vi "createTestObject.vi"(11 "Data in":T1={"Report.lvclass"=refnum, "Norm"="", "last State"=enum."Initialize", "Norm ID"=0, "EMTestCWS500N.lvclass"=refnum, "CEG4500.lvclass"=refnum, "Tektronix RSA5106A.lvclass"=refnum, "erfolgreich"=FALSE, "Device Enum"=enum."emTestCWS500N", "Test Enum"=enum."ESD", "debug"=FALSE, "tab"=enum."Hauptmenü", "ESD Pistol.lvclass"=refnum, "SubPnl Refnum"=refnum, "TabCtl Refnum"=refnum, "ButtonsEinblenden?"=FALSE, "VKey"=enum."ASCII", "last Test"=refnum}) -> (3 "Data out":T1={"Report.lvclass"=refnum, "Norm"="", "last State"=enum."Initialize", "Norm ID"=0, "EMTestCWS500N.lvclass"=refnum, "CEG4500.lvclass"=refnum, "Tektronix RSA5106A.lvclass"=refnum, "erfolgreich"=FALSE, "Device Enum"=enum."emTestCWS500N", "Test Enum"=enum."ESD", "debug"=FALSE, "tab"=enum."Hauptmenü", "ESD Pistol.lvclass"=refnum, "SubPnl Refnum"=refnum, "TabCtl Refnum"=refnum, "ButtonsEinblenden?"=FALSE, "VKey"=enum."ASCII", "last Test"=refnum})   [LabVIEW 2013]
uses:
  Main/controls/Data.ctl
  classes/Datastructure/Report/Report.lvclass
  classes/Devices/emTestCWS500N/EMTestCWS500N.lvclass
  classes/Devices/CEG4500/CEG4500.lvclass
  classes/Devices/Tektronix RSA5106A/Tektronix RSA5106A.lvclass
  ESD Pistol.lvclass
  classes/Datastructure/Test/Test.lvclass
  Main/controls/State.ctl
  classes/Devices/DeviceInterface/Devices.ctl
  classes/Tests/TestInterface/Tests.ctl
  Tabs.ctl
  <vilib>/event_ctls.llb/eventvkey.ctl
  classes/Tests/TestInterface/TestInterface.lvclass
  classes/Devices/DeviceInterface/DeviceInterface.lvclass
  classes/Tests/Stoeraussendung/Stoeraussendung.lvclass
  classes/Tests/Burst/Burst.lvclass
  classes/Tests/Surge/Surge.lvclass
  classes/Tests/Spannungseinbruch/Spannungseinbruch.lvclass
  classes/Tests/HF-Felder/HF-Felder.lvclass
  classes/Tests/ESD/ESD.lvclass
panel:
  out "error out":errorcluster
  in  "error in":errorcluster
types:
  T1 = typedef "Data.ctl" = cluster{"Report.lvclass":refnum<class "Report.lvclass">, "Norm":string, "last State":T2, "Norm ID":i32, "EMTestCWS500N.lvclass":refnum<class "EMTestCWS500N.lvclass">, "CEG4500.lvclass":refnum<class "CEG4500.lvclass">, "Tektronix RSA5106A.lvclass":refnum<class "Tektronix RSA5106A.lvclass">, "erfolgreich":bool, "Device Enum":T3, "Test Enum":T4, "debug":bool, "tab":T5, "ESD Pistol.lvclass":refnum<class "ESD Pistol.lvclass">, "SubPnl Refnum":refnum<vi>, "TabCtl Refnum":refnum<vi>, "ButtonsEinblenden?":bool, "VKey":T6, "last Test":refnum<class "Test.lvclass">}
  T2 = typedef "State.ctl" = enum16{"create Pdf", "edit Report", "load Report", "save Report", "do Test", "CDN Kalibrierung", "enter Report Parameters", "new Test", "Protokoll", "read Tree", "update Tree", "Fehler", "Initialize", "Wait for Event", "Exit"}
  T3 = typedef "Devices.ctl" = enum16{"unbekannt", "ESD Pistol", "Tektronix RSA5106A", "emTestCWS500N", "CEG-4500"}
  T4 = typedef "Tests.ctl" = enum16{"unbekannt", "Störaussendung", "Burst", "ESD", "Surge", "Spannungseinbruch", "HF-Felder"}
  T5 = typedef "Tabs.ctl" = enum32{"Hauptmenü", "Prüfbericht", "Einstellungen"}
  T6 = typedef "eventvkey.ctl" = enum16{"ASCII", "Enter", "Return", "Shift", "Ctrl", "Alt", "Cmd", "Opt", "Caps", "NumLock", "Clear", "Break", "Up", "Down", "Left", "Right", "Insert", "Delete", "Home", "End", "PageUp", "PageDown", "Escape", "Help", "Pause", "ScrollLock", "F1", "F2", "F3", "F4", "F5", "F6", "F7", "F8", "F9", "F10", "F11", "F12", "F13", "F14", "F15", "F16", "F17", "F18", "F19", "F20", "F21", "F22", "F23", "F24", "Play", "VolumeUp", "VolumeDown", "Mute", "Two Byte Char"}
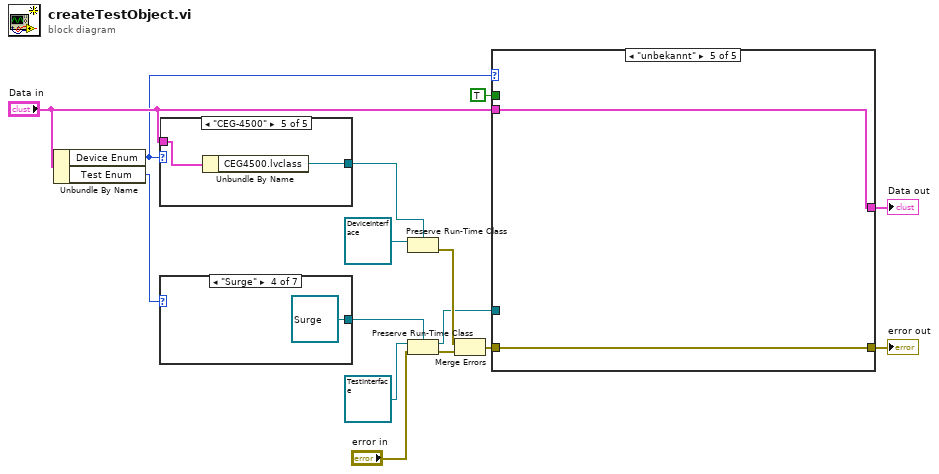
[diagram p0: block diagram]
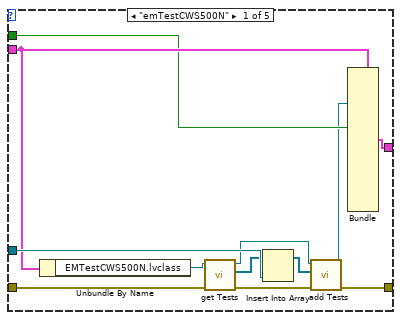
[diagram p2: hidden frame]
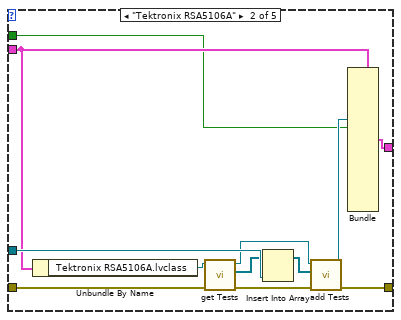
[diagram p3: hidden frame]
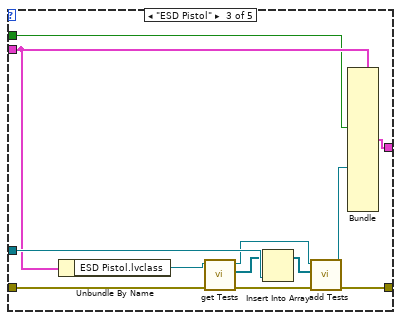
[diagram p4: hidden frame]
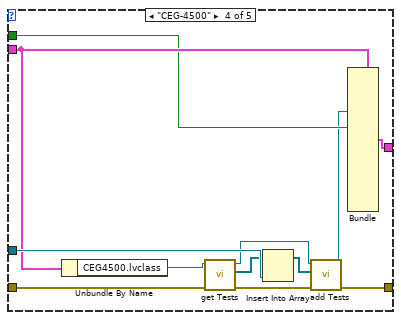
[diagram p5: hidden frame]
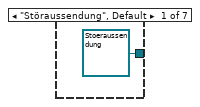
[diagram p6: hidden frame]
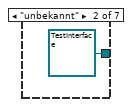
[diagram p7: hidden frame]
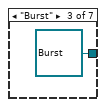
[diagram p8: hidden frame]
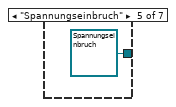
[diagram p9: hidden frame]
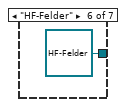
[diagram p10: hidden frame]
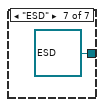
[diagram p11: hidden frame]
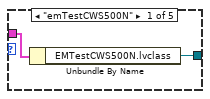
[diagram p12: hidden frame]
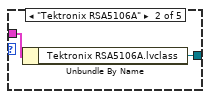
[diagram p13: hidden frame]
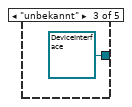
[diagram p14: hidden frame]
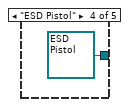
[diagram p15: hidden frame]
diagram:
  n1 = Unbundle By Name("Data in") -> ("Device Enum"=w12:T3, "Test Enum"=w11:T4)
  n2 = case shown="\"CEG-4500\"" w12 {
    tunnel: [w16 w18 refnum<class "DeviceInterface.lvclass"> refnum ("Tektronix RSA5106A.lvclass") refnum<class "ESD Pistol.lvclass"> refnum ("ESD Pistol.lvclass") w22] -> w9
    tunnel: "Data in" -> [w17 w19 _ _ w23]
    frame "emTestCWS500N" {
      n3 = Unbundle By Name(w17) -> ("EMTestCWS500N.lvclass"=w16:refnum<class "EMTestCWS500N.lvclass">)
    }
    frame "Tektronix RSA5106A" {
      n4 = Unbundle By Name(w19) -> ("Tektronix RSA5106A.lvclass"=w18:refnum<class "Tektronix RSA5106A.lvclass">)
    }
    frame "unbekannt" {
    }
    frame "ESD Pistol" {
    }
    frame "CEG-4500" {
      n5 = Unbundle By Name(w23) -> ("CEG4500.lvclass"=w22:refnum<class "CEG4500.lvclass">)
    }
  }
  n6 = case shown="\"Surge\"" w11 {
    tunnel: [refnum<class "Stoeraussendung.lvclass"> refnum ("Störaussendung.lvclass") refnum<class "TestInterface.lvclass"> refnum ("Burst.lvclass") refnum<class "Burst.lvclass"> refnum ("Burst.lvclass") refnum<class "Surge.lvclass"> refnum ("Surge.lvclass") refnum<class "Spannungseinbruch.lvclass"> refnum ("Spannungseinbruch.lvclass") refnum<class "HF-Felder.lvclass"> refnum ("HF-Felder.lvclass") refnum<class "ESD.lvclass"> refnum ("ESD.lvclass")] -> w6
    frame "Störaussendung", Default {
    }
    frame "unbekannt" {
    }
    frame "Burst" {
    }
    frame "Surge" {
    }
    frame "Spannungseinbruch" {
    }
    frame "HF-Felder" {
    }
    frame "ESD" {
    }
  }
  n7 = Preserve Run-Time Class(object in=refnum<class "DeviceInterface.lvclass"> refnum ("DeviceInterface.lvclass"), 2:w9) -> (error out=w8:errorcluster)  [unwired: 1 in, 1 out]
  n8 = Preserve Run-Time Class(object in=refnum<class "TestInterface.lvclass"> refnum ("TestInterface.lvclass"), error in="error in", 2:w6) -> (object out=w3:refnum<class "TestInterface.lvclass">, error out=w7:errorcluster)
  n9 = Merge Errors(w8, w7) -> (w2:errorcluster)
  n10 = case shown="\"unbekannt\"" w12 {
    tunnel: TRUE ("erfolgreich") -> [w32 w43 w56 w68 _]
    tunnel: w3 -> [w42 w54 w66 w78 _]
    tunnel: w2 -> [w41 w53 w65 w77 w80]
    tunnel: [w40 w52 w64 w76 w80] -> w13
    tunnel: [w39 w51 w63 w75 w79] -> w14
    tunnel: "Data in" -> [w38 w50 w62 w74 w79]
    frame "emTestCWS500N" {
      n11 = Unbundle By Name(w38) -> ("EMTestCWS500N.lvclass"=w37:refnum<class "EMTestCWS500N.lvclass">)
      n12 = call-dynamic "get Tests.vi"("error in (no error)"=w41, "DeviceInterface (Eingang)"=w37) -> ("error out"=w33:errorcluster, "Tests"=w36:refnum<class "TestInterface.lvclass">[], "DeviceInterface (Ausgang)"=w34:refnum<class "EMTestCWS500N.lvclass">)  [unwired: 7 in]
      n13 = Insert Into Array(array=w36, new element=w42) -> (w35:refnum<class "TestInterface.lvclass">[])  [unwired: 1 in]
      n14 = call-dynamic "add Tests.vi"("error in (no error)"=w33, "Tests"=w35, "DeviceInterface (Eingang)"=w34) -> ("error out"=w40:errorcluster, "DeviceInterface (Ausgang)"=w31:refnum<class "EMTestCWS500N.lvclass">)  [unwired: 7 in]
      n15 = Bundle(cluster=w38, "EMTestCWS500N.lvclass"=w31, "erfolgreich"=w32) -> (w39:T1)  [unwired: 16 in]
    }
    frame "Tektronix RSA5106A" {
      n16 = Unbundle By Name(w50) -> ("Tektronix RSA5106A.lvclass"=w49:refnum<class "Tektronix RSA5106A.lvclass">)
      n17 = call-dynamic "get Tests.vi"("error in (no error)"=w53, "DeviceInterface (Eingang)"=w49) -> ("error out"=w45:errorcluster, "Tests"=w48:refnum<class "TestInterface.lvclass">[], "DeviceInterface (Ausgang)"=w46:refnum<class "Tektronix RSA5106A.lvclass">)  [unwired: 7 in]
      n18 = Insert Into Array(array=w48, new element=w54) -> (w47:refnum<class "TestInterface.lvclass">[])  [unwired: 1 in]
      n19 = call-dynamic "add Tests.vi"("error in (no error)"=w45, "Tests"=w47, "DeviceInterface (Eingang)"=w46) -> ("error out"=w52:errorcluster, "DeviceInterface (Ausgang)"=w44:refnum<class "Tektronix RSA5106A.lvclass">)  [unwired: 7 in]
      n20 = Bundle(cluster=w50, "Tektronix RSA5106A.lvclass"=w44, "erfolgreich"=w43) -> (w51:T1)  [unwired: 16 in]
    }
    frame "ESD Pistol" {
      n21 = Unbundle By Name(w62) -> ("ESD Pistol.lvclass"=w61:refnum<class "ESD Pistol.lvclass">)
      n22 = call-dynamic "get Tests.vi"("error in (no error)"=w65, "DeviceInterface (Eingang)"=w61) -> ("error out"=w57:errorcluster, "Tests"=w60:refnum<class "TestInterface.lvclass">[], "DeviceInterface (Ausgang)"=w58:refnum<class "ESD Pistol.lvclass">)  [unwired: 7 in]
      n23 = Insert Into Array(array=w60, new element=w66) -> (w59:refnum<class "TestInterface.lvclass">[])  [unwired: 1 in]
      n24 = call-dynamic "add Tests.vi"("error in (no error)"=w57, "Tests"=w59, "DeviceInterface (Eingang)"=w58) -> ("error out"=w64:errorcluster, "DeviceInterface (Ausgang)"=w55:refnum<class "ESD Pistol.lvclass">)  [unwired: 7 in]
      n25 = Bundle(cluster=w62, "erfolgreich"=w56, "ESD Pistol.lvclass"=w55) -> (w63:T1)  [unwired: 16 in]
    }
    frame "CEG-4500" {
      n26 = Unbundle By Name(w74) -> ("CEG4500.lvclass"=w73:refnum<class "CEG4500.lvclass">)
      n27 = call-dynamic "get Tests.vi"("error in (no error)"=w77, "DeviceInterface (Eingang)"=w73) -> ("error out"=w69:errorcluster, "Tests"=w72:refnum<class "TestInterface.lvclass">[], "DeviceInterface (Ausgang)"=w70:refnum<class "CEG4500.lvclass">)  [unwired: 7 in]
      n28 = Insert Into Array(array=w72, new element=w78) -> (w71:refnum<class "TestInterface.lvclass">[])  [unwired: 1 in]
      n29 = call-dynamic "add Tests.vi"("error in (no error)"=w69, "Tests"=w71, "DeviceInterface (Eingang)"=w70) -> ("error out"=w76:errorcluster, "DeviceInterface (Ausgang)"=w67:refnum<class "CEG4500.lvclass">)  [unwired: 7 in]
      n30 = Bundle(cluster=w74, "CEG4500.lvclass"=w67, "erfolgreich"=w68) -> (w75:T1)  [unwired: 16 in]
    }
    frame "unbekannt" {
    }
  }
  "Data out" <- w14
  "error out" <- w13
